vi "MatrixSwitch.vi"(8 "error in (no error)":errorcluster, 10 "Action":T1(ring), 11 "LXIPXISwitching in":refnum<class "LXIPXISwitching.lvclass">) -> (0 "error out":errorcluster, 2 "Continue?":bool, 3 "LXIPXISwitching out":refnum<class "LXIPXISwitching.lvclass">)   [LabVIEW 2019, in "LXIPXISwitching.lvclass"]
uses:
  LXIPXISwitching.lvclass
  InstrumentSetup.vi
  InstrControl.lvclass
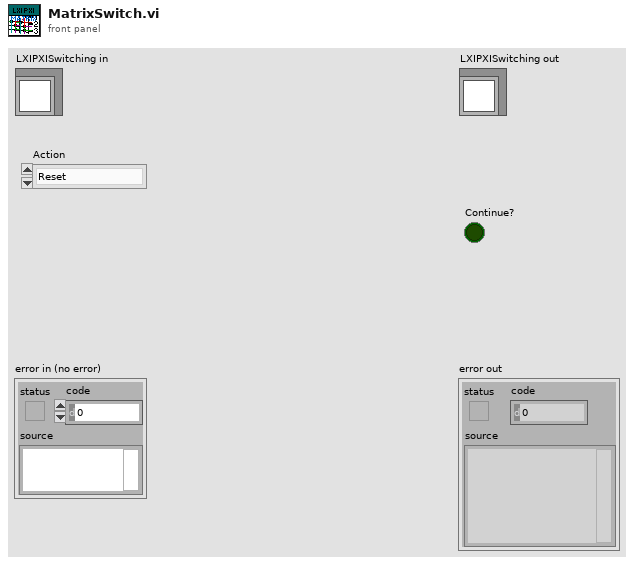
[diagram p1: front panel]
types:
  T1 = enum16{"Reset", "Ground", "Striptest Bias", "Striptest SMU", "Striptest LCR", "IV", "CV", "Interstrip Cap", "Interstrip Res", "PTP", "Implant Resistance", "Metal Resistance", "Coupling Capacitance"}
  T2 = cluster{"MUX":string, "Matrix":string, "Breadboard":string, "LXIPXI Switching":refnum<class "LXIPXISwitching.lvclass">, "MUX PN":string, "Matrix  PN":string, "Breadboard PN":string, "MUX ID":string, "Matrix ID":string, "Breadboard ID":string, "LCR?":bool, "SMU?":bool}
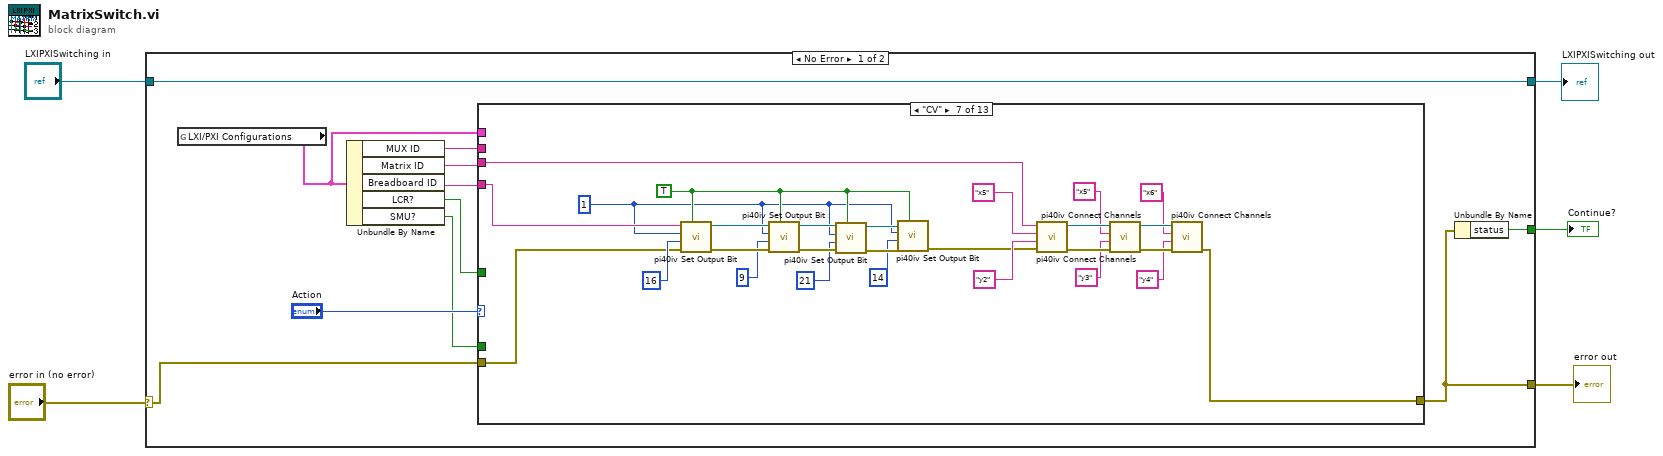
[diagram p0: block diagram]
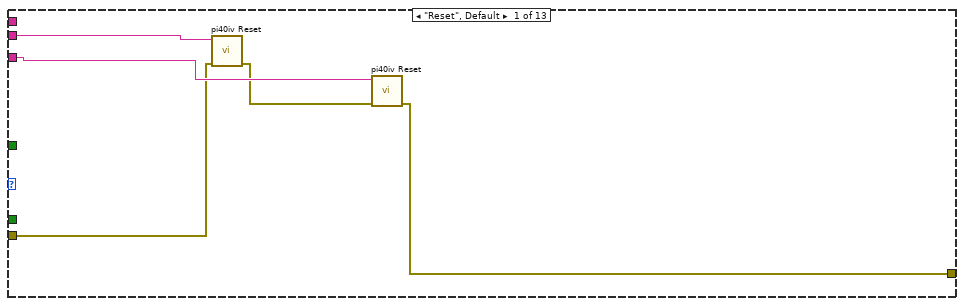
[diagram p2: hidden frame]
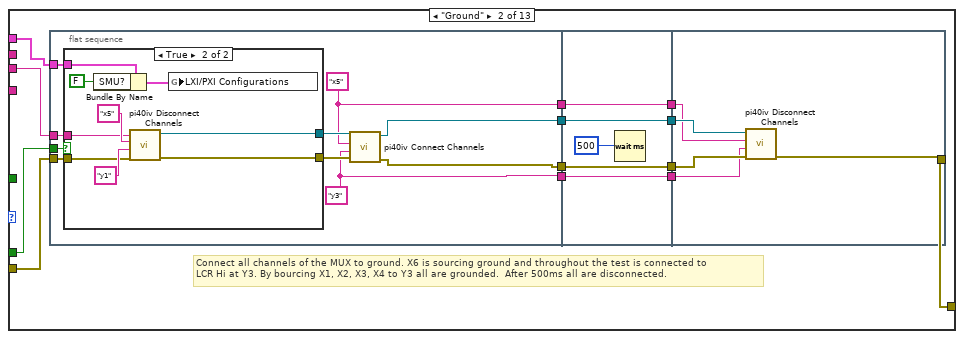
[diagram p3: hidden frame]
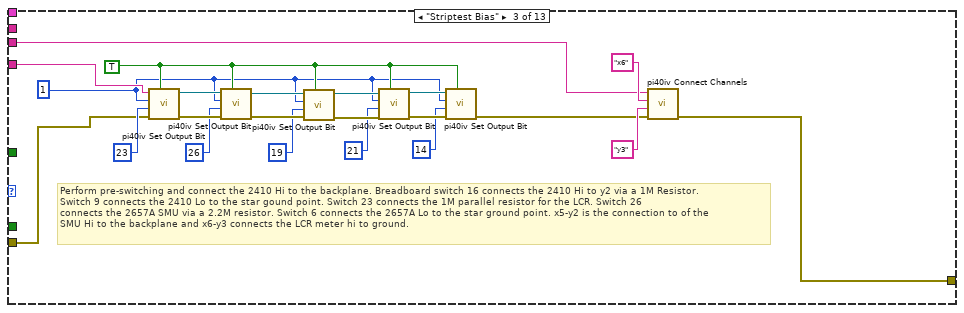
[diagram p5: hidden frame]
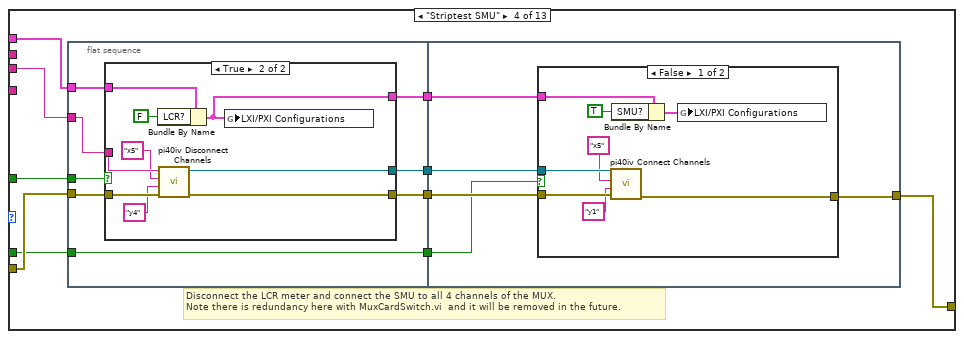
[diagram p6: hidden frame]
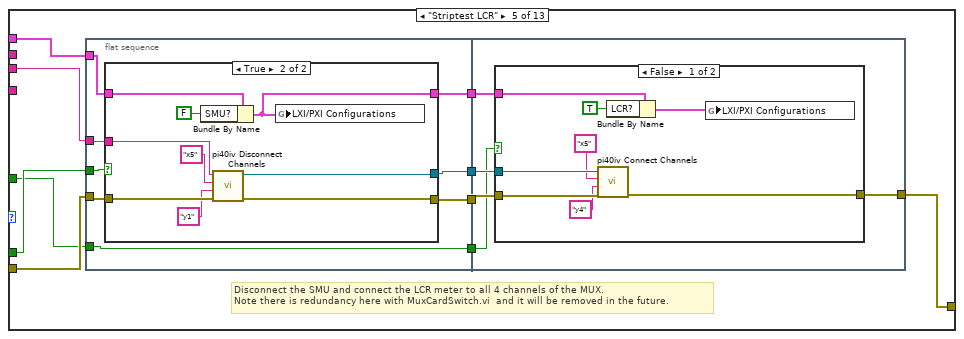
[diagram p9: hidden frame]
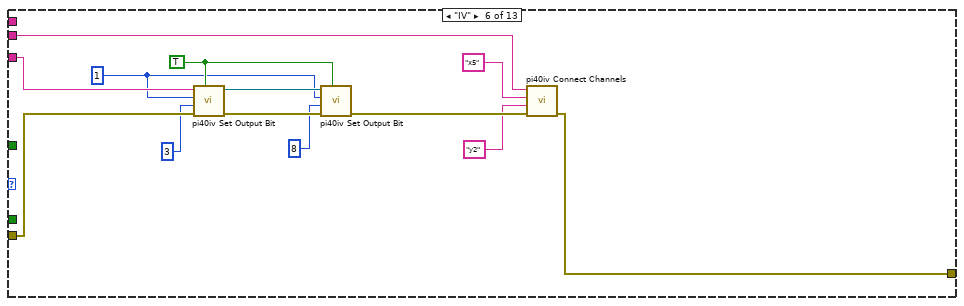
[diagram p12: hidden frame]
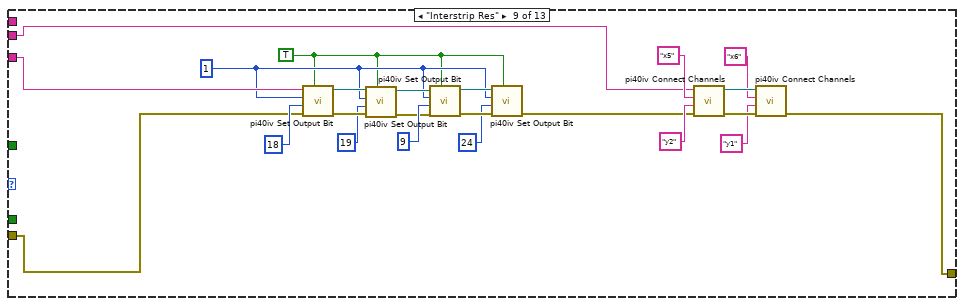
[diagram p14: hidden frame]
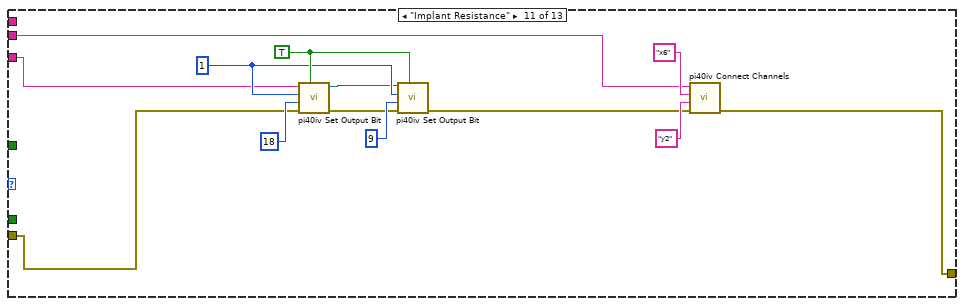
[diagram p16: hidden frame]
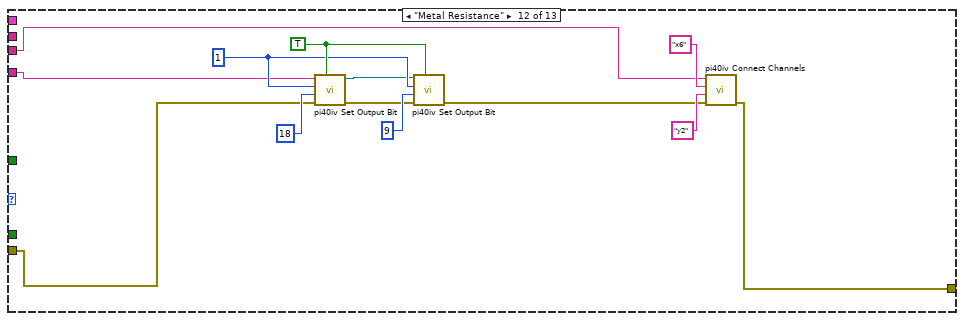
[diagram p17: hidden frame]
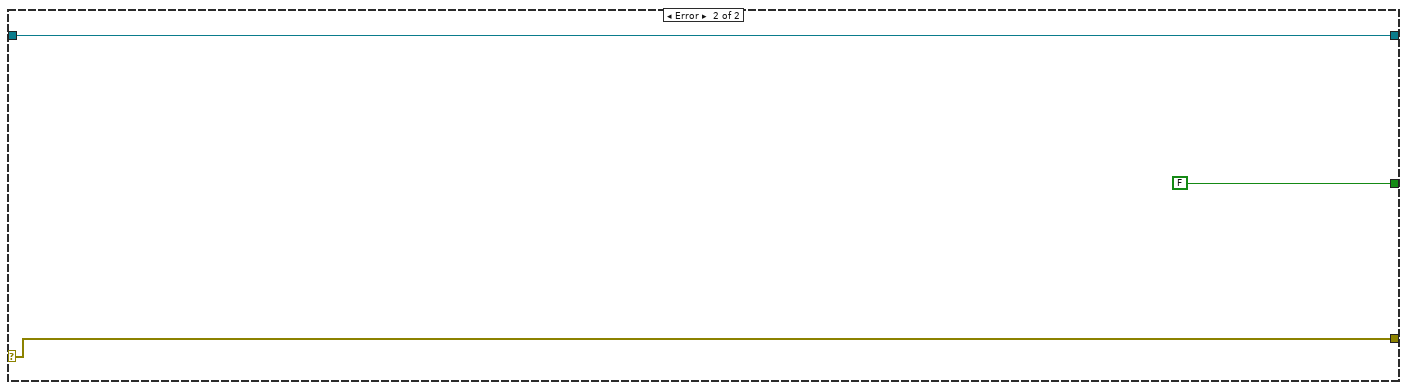
[diagram p19: hidden frame]
diagram:
  n1 = case shown="No Error" "error in (no error)" {
    selector: "error in (no error)" -> [w13 w270]
    tunnel: [w15 w268] -> w3
    tunnel: "LXIPXISwitching in" -> [w15 w268]
    tunnel: [w14 FALSE ("status")] -> w2
    tunnel: [w10 w270] -> w1
    frame No Error {
      n2 = global read "InstrumentSetup.vi" "LXI/PXI Configurations"() -> (w6:T2)
      n3 = Unbundle By Name(w6) -> ("MUX ID"=w9:string, "Matrix ID"=w12:string, "Breadboard ID"=w11:string, "LCR?"=w8:bool, "SMU?"=w7:bool)
      n4 = case shown="\"CV\"" "Action" {
        tunnel: w13 -> [w19 w33 w77 w95 w138 w184 w207 w216 w231 w240 w246 w256 w267]
        tunnel: w12 -> [w21 w34 w75 w97 w139 w187 w209 _ w218 _ w247 w254 _]
        tunnel: w11 -> [w20 _ w76 _ _ w186 w208 _ w229 _ w245 w257 _]
        tunnel: [w17 w29 w80 w93 w137 w181 w202 w216 w230 w240 w241 w255 w267] -> w10
        tunnel: w9 -> [_ _ _ _ _ _ _ _ _ _ _ _ _]
        tunnel: w8 -> [_ _ _ w92 w135 _ _ _ _ _ _ _ _]
        tunnel: w7 -> [_ w25 _ w90 w136 _ _ _ _ _ _ _ _]
        tunnel: w6 -> [_ w24 _ w89 w133 _ _ _ _ _ _ _ _]
        frame "Reset", Default {
          n5 = call <instrlib>:"pi40iv Reset.vi"("error in (no error)"=w19, "instrument handle"=w21) -> ("error out"=w18:errorcluster)  [unwired: 8 in, 1 out]
          n6 = call <instrlib>:"pi40iv Reset.vi"("error in (no error)"=w18, "instrument handle"=w20) -> ("error out"=w17:errorcluster)  [unwired: 8 in, 1 out]
        }
        frame "Ground" {
          # "Connect all channels of the MUX to ground. X6 is sourcing ground and throughout the test is connected to \nLCR Hi at Y3. By bourcing X1, X2, X3, X4 to Y3 all are grounded.  After 500ms all are disconnected."
          n7 = flat-sequence {
            tunnel: w34 -> [w41]
            tunnel: w33 -> [w44]
            tunnel: [w37] -> w30
            tunnel: [w36] -> w28
            tunnel: [w38] -> w26
            tunnel: w25 -> [w40]
            tunnel: w24 -> [w39]
            tunnel: [w35] -> w22
            tunnel: [w59] -> w32
            tunnel: [w58] -> w31
            tunnel: w30 -> [w58]
            tunnel: w28 -> [w59]
            tunnel: [w57] -> w27
            tunnel: w26 -> [w57]
            tunnel: [w56] -> w23
            tunnel: w22 -> [w56]
            tunnel: w32 -> [w64]
            tunnel: w31 -> [w65]
            tunnel: [w62] -> w29
            tunnel: w27 -> [w63]
            tunnel: w23 -> [w61]
            frame #0 {
              w38 = "y3" ("channel 2")
              w35 = "x5" ("channel 1")
              n8 = case shown="True" w40 {
                tunnel: w44 -> [w45 w53]
                tunnel: [w45 w48] -> w43
                tunnel: [w46 w47] -> w42
                tunnel: w41 -> [w46 w52]
                tunnel: w39 -> [_ w49]
                frame False {
                }
                frame True {
                  n9 = Bundle By Name(cluster=w49, "SMU?"=FALSE) -> (w51:T2)
                  n10 = call <instrlib>:"pi40iv Disconnect Channels.vi"("error in (no error)"=w53, "channel 2"="y1", "channel 1"="x5", "instrument handle"=w52) -> ("error out"=w48:errorcluster, "instrument handle out"=w47:refnum<k15>)  [unwired: 6 in]
                  n11 = global write "InstrumentSetup.vi" "LXI/PXI Configurations"(w51) -> ()
                }
              }
              n12 = call <instrlib>:"pi40iv Connect Channels.vi"("error in (no error)"=w43, "channel 2"=w38, "channel 1"=w35, "instrument handle"=w42) -> ("error out"=w37:errorcluster, "instrument handle out"=w36:refnum<k15>)  [unwired: 6 in]
            }
            frame #1 {
              n13 = Wait (ms)(milliseconds to wait=u32 500) -> ()  [unwired: 1 out]
            }
            frame #2 {
              n14 = call <instrlib>:"pi40iv Disconnect Channels.vi"("error in (no error)"=w65, "channel 2"=w63, "channel 1"=w61, "instrument handle"=w64) -> ("error out"=w62:errorcluster)  [unwired: 6 in, 1 out]
            }
          }
        }
        frame "Striptest Bias" {
          w66 = u32 1 ("output sub number")
          w71 = TRUE ("state")
          # "Perform pre-switching and connect the 2410 Hi to the backplane. Breadboard switch 16 connects the 2410 Hi to y2 via a 1M Resistor.\nSwitch 9 connects the 2410 Lo to the star gound point. Switch 23 connects the 1M parallel resistor for the LCR. Switch 26 \nconnects the 2657A SMU via a 2.2M resistor. Switch 6 connects the 2657A Lo to the star ground point. x5-y2 is the connection to of the \nSMU Hi to the backplane and x6-y3 connects the LCR meter hi to ground."
          n15 = call <instrlib>:"pi40iv Set Output Bit.vi"("state"=w71, "error in (no error)"=w77, "bit number"=u32 23, "output sub number"=w66, "instrument handle"=w76) -> ("error out"=w86:errorcluster, "instrument handle out"=w85:refnum<k15>)  [unwired: 5 in]
          n16 = call <instrlib>:"pi40iv Set Output Bit.vi"("state"=w71, "error in (no error)"=w86, "bit number"=u32 26, "output sub number"=w66, "instrument handle"=w85) -> ("error out"=w83:errorcluster, "instrument handle out"=w82:refnum<k15>)  [unwired: 5 in]
          n17 = call <instrlib>:"pi40iv Set Output Bit.vi"("state"=w71, "error in (no error)"=w83, "bit number"=u32 19, "output sub number"=w66, "instrument handle"=w82) -> ("error out"=w74:errorcluster, "instrument handle out"=w68:refnum<k15>)  [unwired: 5 in]
          n18 = call <instrlib>:"pi40iv Set Output Bit.vi"("state"=w71, "error in (no error)"=w74, "bit number"=u32 21, "output sub number"=w66, "instrument handle"=w68) -> ("error out"=w73:errorcluster, "instrument handle out"=w67:refnum<k15>)  [unwired: 5 in]
          n19 = call <instrlib>:"pi40iv Set Output Bit.vi"("state"=w71, "error in (no error)"=w73, "bit number"=u32 14, "output sub number"=w66, "instrument handle"=w67) -> ("error out"=w72:errorcluster)  [unwired: 5 in, 1 out]
          n20 = call <instrlib>:"pi40iv Connect Channels.vi"("error in (no error)"=w72, "channel 2"="y3", "channel 1"="x6", "instrument handle"=w75) -> ("error out"=w80:errorcluster)  [unwired: 6 in, 1 out]
        }
        frame "Striptest SMU" {
          # "Disconnect the LCR meter and connect the SMU to all 4 channels of the MUX.\nNote there is redundancy here with MuxCardSwitch.vi  and it will be removed in the future."
          n21 = flat-sequence {
            tunnel: w97 -> [w105]
            tunnel: [w103] -> w96
            tunnel: w95 -> [w104]
            tunnel: [w102] -> w94
            tunnel: w92 -> [w101]
            tunnel: [w100] -> w91
            tunnel: w90 -> [w100]
            tunnel: w89 -> [w99]
            tunnel: [w98] -> w88
            tunnel: w96 -> [w122]
            tunnel: w94 -> [w121]
            tunnel: [w120] -> w93
            tunnel: w91 -> [w119]
            tunnel: w88 -> [w118]
            frame #0 {
              n22 = case shown="True" w101 {
                tunnel: w105 -> [w108 w117]
                tunnel: w104 -> [w107 w116]
                tunnel: [w108 w109] -> w103
                tunnel: [w107 w110] -> w102
                tunnel: w99 -> [w106 w113]
                tunnel: [w106 w111] -> w98
                frame False {
                }
                frame True {
                  n23 = Bundle By Name(cluster=w113, "LCR?"=FALSE) -> (w111:T2)
                  n24 = call <instrlib>:"pi40iv Disconnect Channels.vi"("error in (no error)"=w116, "channel 2"="y4", "channel 1"="x5", "instrument handle"=w117) -> ("error out"=w110:errorcluster, "instrument handle out"=w109:refnum<k15>)  [unwired: 6 in]
                  n25 = global write "InstrumentSetup.vi" "LXI/PXI Configurations"(w111) -> ()
                }
              }
            }
            frame #1 {
              n26 = case shown="False" w119 {
                tunnel: w122 -> [w130 _]
                tunnel: w121 -> [w129 w131]
                tunnel: [w123 w131] -> w120
                tunnel: w118 -> [w126 _]
                frame False {
                  n27 = call <instrlib>:"pi40iv Connect Channels.vi"("error in (no error)"=w129, "channel 2"="y1", "channel 1"="x5", "instrument handle"=w130) -> ("error out"=w123:errorcluster)  [unwired: 6 in, 1 out]
                  n28 = Bundle By Name(cluster=w126, "SMU?"=TRUE) -> (w125:T2)
                  n29 = global write "InstrumentSetup.vi" "LXI/PXI Configurations"(w125) -> ()
                }
                frame True {
                }
              }
            }
          }
        }
        frame "Striptest LCR" {
          # "Disconnect the SMU and connect the LCR meter to all 4 channels of the MUX.\nNote there is redundancy here with MuxCardSwitch.vi  and it will be removed in the future."
          n30 = flat-sequence {
            tunnel: w139 -> [w149]
            tunnel: [w147] -> w141
            tunnel: w138 -> [w148]
            tunnel: [w146] -> w140
            tunnel: w136 -> [w145]
            tunnel: w135 -> [w144]
            tunnel: [w144] -> w134
            tunnel: w133 -> [w143]
            tunnel: [w142] -> w132
            tunnel: w141 -> [w166]
            tunnel: w140 -> [w165]
            tunnel: [w164] -> w137
            tunnel: w134 -> [w163]
            tunnel: w132 -> [w162]
            frame #0 {
              n31 = case shown="True" w145 {
                tunnel: w149 -> [w152 w161]
                tunnel: w148 -> [w151 w160]
                tunnel: [w152 w153] -> w147
                tunnel: [w151 w154] -> w146
                tunnel: w143 -> [w150 w157]
                tunnel: [w150 w155] -> w142
                frame False {
                }
                frame True {
                  n32 = Bundle By Name(cluster=w157, "SMU?"=FALSE) -> (w155:T2)
                  n33 = call <instrlib>:"pi40iv Disconnect Channels.vi"("error in (no error)"=w160, "channel 2"="y1", "channel 1"="x5", "instrument handle"=w161) -> ("error out"=w154:errorcluster, "instrument handle out"=w153:refnum<k15>)  [unwired: 6 in]
                  n34 = global write "InstrumentSetup.vi" "LXI/PXI Configurations"(w155) -> ()
                }
              }
            }
            frame #1 {
              n35 = case shown="False" w163 {
                tunnel: w166 -> [w174 _]
                tunnel: w165 -> [w173 w175]
                tunnel: [w167 w175] -> w164
                tunnel: w162 -> [w170 _]
                frame False {
                  n36 = call <instrlib>:"pi40iv Connect Channels.vi"("error in (no error)"=w173, "channel 2"="y4", "channel 1"="x5", "instrument handle"=w174) -> ("error out"=w167:errorcluster)  [unwired: 6 in, 1 out]
                  n37 = Bundle By Name(cluster=w170, "LCR?"=TRUE) -> (w168:T2)
                  n38 = global write "InstrumentSetup.vi" "LXI/PXI Configurations"(w168) -> ()
                }
                frame True {
                }
              }
            }
          }
        }
        frame "IV" {
          w176 = u32 1 ("output sub number")
          w188 = TRUE ("state")
          n39 = call <instrlib>:"pi40iv Set Output Bit.vi"("state"=w188, "error in (no error)"=w184, "bit number"=u32 3, "output sub number"=w176, "instrument handle"=w186) -> ("error out"=w183:errorcluster, "instrument handle out"=w185:refnum<k15>)  [unwired: 5 in]
          n40 = call <instrlib>:"pi40iv Set Output Bit.vi"("state"=w188, "error in (no error)"=w183, "bit number"=u32 8, "output sub number"=w176, "instrument handle"=w185) -> ("error out"=w182:errorcluster)  [unwired: 5 in, 1 out]
          n41 = call <instrlib>:"pi40iv Connect Channels.vi"("error in (no error)"=w182, "channel 2"="y2", "channel 1"="x5", "instrument handle"=w187) -> ("error out"=w181:errorcluster)  [unwired: 6 in, 1 out]
        }
        frame "CV" {
          w191 = u32 1 ("output sub number")
          w192 = TRUE ("state")
          n42 = call <instrlib>:"pi40iv Set Output Bit.vi"("state"=w192, "error in (no error)"=w207, "bit number"=u32 16, "output sub number"=w191, "instrument handle"=w208) -> ("error out"=w214:errorcluster, "instrument handle out"=w215:refnum<k15>)  [unwired: 5 in]
          n43 = call <instrlib>:"pi40iv Set Output Bit.vi"("state"=w192, "error in (no error)"=w214, "bit number"=u32 9, "output sub number"=w191, "instrument handle"=w215) -> ("error out"=w197:errorcluster, "instrument handle out"=w194:refnum<k15>)  [unwired: 5 in]
          n44 = call <instrlib>:"pi40iv Set Output Bit.vi"("state"=w192, "error in (no error)"=w197, "bit number"=u32 21 ("output sub number"), "output sub number"=w191, "instrument handle"=w194) -> ("error out"=w196:errorcluster, "instrument handle out"=w193:refnum<k15>)  [unwired: 5 in]
          n45 = call <instrlib>:"pi40iv Set Output Bit.vi"("state"=w192, "error in (no error)"=w196, "bit number"=u32 14, "output sub number"=w191, "instrument handle"=w193) -> ("error out"=w195:errorcluster)  [unwired: 5 in, 1 out]
          n46 = call <instrlib>:"pi40iv Connect Channels.vi"("error in (no error)"=w195, "channel 2"="y2", "channel 1"="x5", "instrument handle"=w209) -> ("error out"=w204:errorcluster, "instrument handle out"=w206:refnum<k15>)  [unwired: 6 in]
          n47 = call <instrlib>:"pi40iv Connect Channels.vi"("error in (no error)"=w204, "channel 2"="y3", "channel 1"="x5", "instrument handle"=w206) -> ("error out"=w203:errorcluster, "instrument handle out"=w205:refnum<k15>)  [unwired: 6 in]
          n48 = call <instrlib>:"pi40iv Connect Channels.vi"("error in (no error)"=w203, "channel 2"="y4", "channel 1"="x6", "instrument handle"=w205) -> ("error out"=w202:errorcluster)  [unwired: 6 in, 1 out]
        }
        frame "Interstrip Cap" {
          # "To be done..."
        }
        frame "Interstrip Res" {
          w220 = u32 1 ("output sub number")
          w217 = TRUE ("state")
          n49 = call <instrlib>:"pi40iv Set Output Bit.vi"("state"=w217, "error in (no error)"=w231, "bit number"=u32 18, "output sub number"=w220, "instrument handle"=w229) -> ("error out"=w228:errorcluster, "instrument handle out"=w225:refnum<k15>)  [unwired: 5 in]
          n50 = call <instrlib>:"pi40iv Set Output Bit.vi"("state"=w217, "error in (no error)"=w228, "bit number"=u32 19, "output sub number"=w220, "instrument handle"=w225) -> ("error out"=w227:errorcluster, "instrument handle out"=w224:refnum<k15>)  [unwired: 5 in]
          n51 = call <instrlib>:"pi40iv Set Output Bit.vi"("state"=w217, "error in (no error)"=w227, "bit number"=u32 9, "output sub number"=w220, "instrument handle"=w224) -> ("error out"=w223:errorcluster, "instrument handle out"=w222:refnum<k15>)  [unwired: 5 in]
          n52 = call <instrlib>:"pi40iv Set Output Bit.vi"("state"=w217, "error in (no error)"=w223, "bit number"=u32 24, "output sub number"=w220, "instrument handle"=w222) -> ("error out"=w219:errorcluster)  [unwired: 5 in, 1 out]
          n53 = call <instrlib>:"pi40iv Connect Channels.vi"("error in (no error)"=w219, "channel 2"="y2", "channel 1"="x5", "instrument handle"=w218) -> ("error out"=w236:errorcluster, "instrument handle out"=w237:refnum<k15>)  [unwired: 6 in]
          n54 = call <instrlib>:"pi40iv Connect Channels.vi"("error in (no error)"=w236, "channel 2"="y1", "channel 1"="x6", "instrument handle"=w237) -> ("error out"=w230:errorcluster)  [unwired: 6 in, 1 out]
        }
        frame "PTP" {
        }
        frame "Implant Resistance" {
          w248 = u32 1 ("output sub number")
          w249 = TRUE ("state")
          n55 = call <instrlib>:"pi40iv Set Output Bit.vi"("state"=w249, "error in (no error)"=w246, "bit number"=u32 18, "output sub number"=w248, "instrument handle"=w245) -> ("error out"=w243:errorcluster, "instrument handle out"=w244:refnum<k15>)  [unwired: 5 in]
          n56 = call <instrlib>:"pi40iv Set Output Bit.vi"("state"=w249, "error in (no error)"=w243, "bit number"=u32 9, "output sub number"=w248, "instrument handle"=w244) -> ("error out"=w242:errorcluster)  [unwired: 5 in, 1 out]
          n57 = call <instrlib>:"pi40iv Connect Channels.vi"("error in (no error)"=w242, "channel 2"="y2", "channel 1"="x6", "instrument handle"=w247) -> ("error out"=w241:errorcluster)  [unwired: 6 in, 1 out]
        }
        frame "Metal Resistance" {
          w261 = u32 1 ("output sub number")
          w262 = TRUE ("state")
          n58 = call <instrlib>:"pi40iv Set Output Bit.vi"("state"=w262, "error in (no error)"=w256, "bit number"=u32 18, "output sub number"=w261, "instrument handle"=w257) -> ("error out"=w259:errorcluster, "instrument handle out"=w260:refnum<k15>)  [unwired: 5 in]
          n59 = call <instrlib>:"pi40iv Set Output Bit.vi"("state"=w262, "error in (no error)"=w259, "bit number"=u32 9, "output sub number"=w261, "instrument handle"=w260) -> ("error out"=w258:errorcluster)  [unwired: 5 in, 1 out]
          n60 = call <instrlib>:"pi40iv Connect Channels.vi"("error in (no error)"=w258, "channel 2"="y2", "channel 1"="x6", "instrument handle"=w254) -> ("error out"=w255:errorcluster)  [unwired: 6 in, 1 out]
        }
        frame "Coupling Capacitance" {
        }
      }
      n61 = Unbundle By Name(w10) -> ("status"=w14:bool)
    }
    frame Error {
    }
  }
  "error out" <- w1
  "LXIPXISwitching out" <- w3
  "Continue?" <- w2
